vi "Update Chnl Setting.vi"(8 "error in (no error)":errorcluster, 11 "BME_DG_Chnl in":refnum<class "BME_DG_Chnl.lvclass">) -> (0 "error out":errorcluster, 3 "BME_DG_Chnl out":refnum<class "BME_DG_Chnl.lvclass">)   [LabVIEW 2009, in "BME_DG_Chnl.lvclass"]
uses:
  BME_DG_Chnl.lvclass
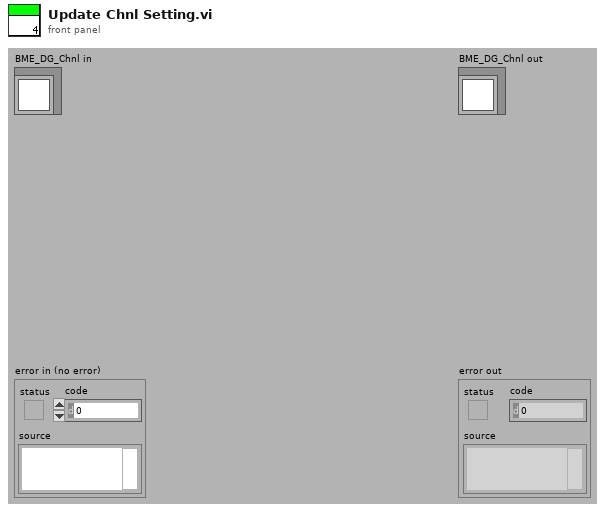
[diagram p1: front panel]
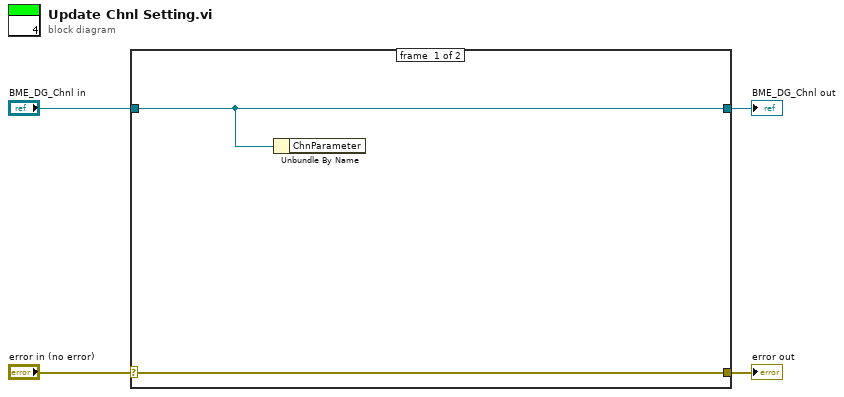
[diagram p0: block diagram]
diagram:
  n1 = case shown="No Error" "error in (no error)" {
    selector: "error in (no error)" -> [w6 w8]
    tunnel: [w6 w8] -> w3
    tunnel: [w5 w7] -> w1
    tunnel: "BME_DG_Chnl in" -> [w5 w7]
    frame #0 {
      n2 = Unbundle By Name(w5) -> ()  [unwired: 1 out]
    }
    frame #1 {
    }
  }
  "error out" <- w3
  "BME_DG_Chnl out" <- w1
